vi "RVC Lane Change.vi"() -> ()   [LabVIEW 2013]
uses:
  <vilib>/Simulation/Scripting/Companion Diagram/SimConfigNode/SimParams.ctl
  <vilib>/Simulation/Scripting/Companion Diagram/SimConfigNode/_simSolvers.ctl
  <vilib>/Simulation/Implementation/Shared/SIMSCR Execution Mode.ctl
  <vilib>/Simulation/Param Hierarchy/Typedefs/SIMPH Param Control Actions.ctl
  <vilib>/Simulation/Scripting/Editor Utilities/SIM subVI tag data.ctl
  <vilib>/Simulation/Scripting/Editor Utilities/SIM subVI execution type.ctl
  <vilib>/Simulation/Implementation/Shared/NILVSim_ParamChanged.vi
  <vilib>/Simulation/Implementation/Shared/NILVSIM_BeginStep.vi
  <vilib>/Simulation/Utility/Implementation/SIM Time.vi
  <vilib>/Simulation/LookUpTables/Implementation/NILVSim LUT 1D.llb/SIM LUT 1D (scalar).vi
  <vilib>/Simulation/Utility/Implementation/NILVSim Collector.llb/SIM Collector (scalar).vi
  <vilib>/Simulation/Implementation/Shared/SIM Fire Discrete SubVI.vi
  <vilib>/Simulation/Implementation/Shared/NILVSim_Manager.vi
  <vilib>/Simulation/Implementation/Shared/NILVSim_FinalizeModel.vi
  <vilib>/Simulation/Utility/Implementation/NILVSim Collector.llb/NILVSim Collector core (scalar).vi
  <vilib>/Simulation/Implementation/Shared/SIM Fire Discrete SubVI (Core).vi
  <vilib>/Simulation/Implementation/Shared/SIM Unbundle Sim Info.vi
  <vilib>/Utility/error.llb/Clear Errors.vi
  <vilib>/Simulation/Implementation/Shared/NILVSim_GetModelError.vi
  <vilib>/Simulation/Implementation/Shared/SIM Bundle Sim Info.vi
  <vilib>/Simulation/Implementation/Shared/SIMSH Read Queue.vi
  <vilib>/Simulation/Implementation/Shared/NILVSim_Initialize.vi
  <vilib>/Simulation/Utility/Implementation/NILVSim Get Time and IsAcceptedStep.vi
  subVIs/2D Animation.vi
  <vilib>/Simulation/Scripting/Companion Diagram/SimConfigNode/SimDog.xnode
  SIM Bicycle.vi
  <vilib>/Simulation/Implementation/XNodeFramework/SimXNode/SimX.xnode
  <vilib>/Simulation/Implementation/Shared/NI_SIM_Implementation.lvlib
panel:
  out "Map Floor":picture
  out "alpha":cluster{"Time":dbl[], "Signal":dbl[]}(graph)
  out "theta":cluster{"Time":dbl[], "Signal":dbl[]}(graph)
  out "y position":cluster{"Time":dbl[], "Signal":dbl[]}(graph)
  out "XY Graph":cluster{"Time":dbl[], "Signal":dbl[]}(graph)
  in  "velocity":dbl(slide)=0.9795918367346939 scale=0.0..1.0
  # "Overview: This describe how to use the bycicle model to...\nInstructions:\n1. Run the VI"
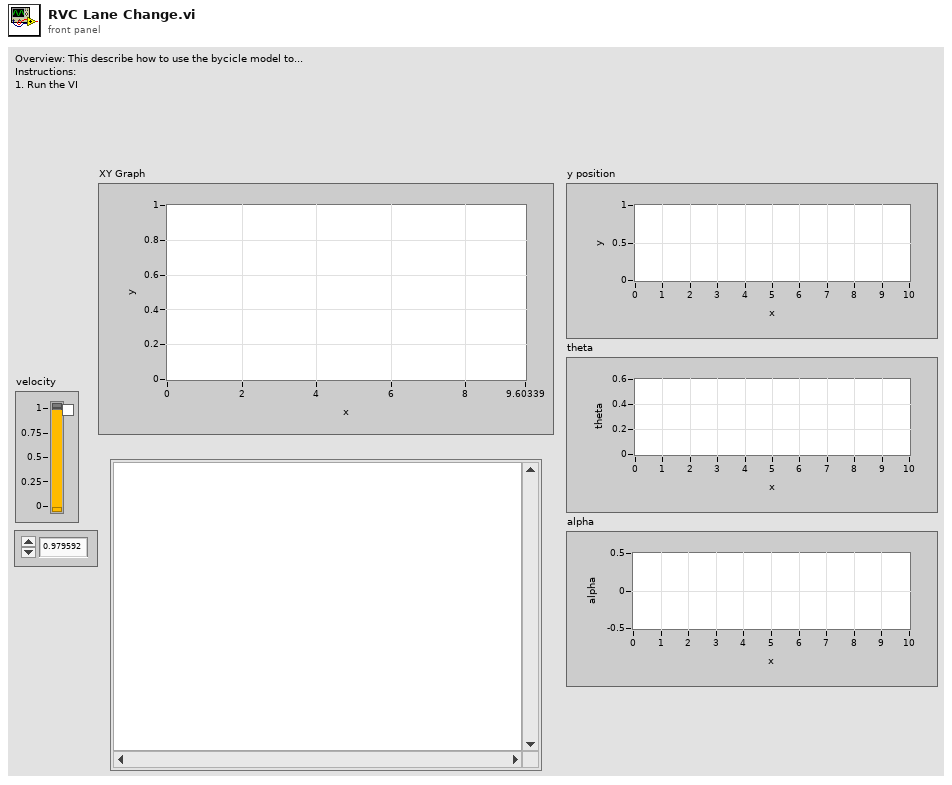
[diagram p1: front panel]
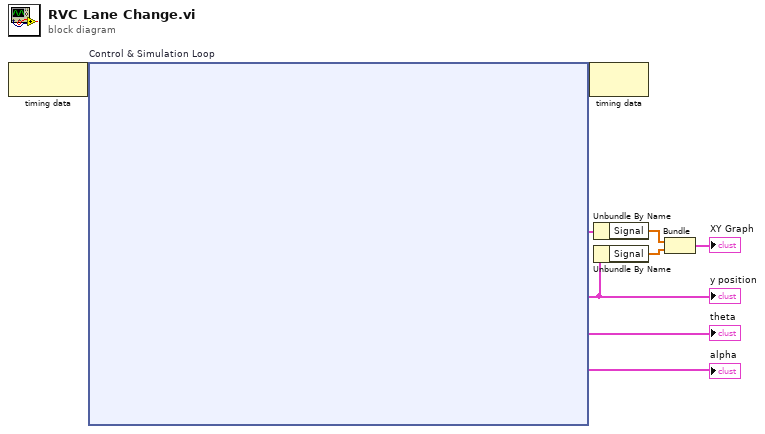
[diagram p0: block diagram]
diagram:
  n1 = node-c288() -> (w9:variant)  [unwired: 1 in]
  n2 = node-c254 "Control & Simulation Loop"(w9) -> (w8:variant, w4:cluster{"Time":dbl[], "Signal":dbl[]}, w3:cluster{"Time":dbl[], "Signal":dbl[]}, →"theta":cluster{"Time":dbl[], "Signal":dbl[]}, →"alpha":cluster{"Time":dbl[], "Signal":dbl[]})
  "y position" <- w3
  n3 = node-c288(w8) -> ()  [unwired: 1 out]
  n4 = Unbundle By Name(w4) -> ("Signal"=w7:dbl[])
  n5 = Unbundle By Name ("Unbundle By Name 2")(w3) -> ("Signal"=w6:dbl[])
  n6 = Bundle("Signal"=w7, "Signal"=w6) -> (→"XY Graph":cluster{"Signal":dbl[], "Signal":dbl[]})  [unwired: 1 in]
